vi "Generate Random Filename.vi"() -> (0 "Random Filename":string)   [LabVIEW 2022 SP3]
doc: "This VI generates a random filename. The random filename is to be used as a temporary filename, while the new VI or CTL is programmatically inserted and moved inside a LabVIEW Project, Library or Class. \n\nThe random temporary name makes it possible for the final name to be the same as another filename that already exists in the project, in a different virtual folder. (avoids name clashes)\n\nThe random filenames are sequences of 16 random lowercase characters. This makes filename clashes virtually impossible. There are 26 letters in the English alphabet, sp there are 26^16 possible 16-letter sequences.\n\nPerformance: This VI is inlined to increase performance"
uses:
  ASCII Character Type.ctl
  Generate Random ASCII Character.vi
  <vilib>/numeric/Random Number (Range).vi
  <vilib>/numeric/Random Number (Range) U64.vi
  <vilib>/numeric/sub_Random U32.vi
panel:
  # "Development\ncontrols/indicators useful for development and testing, but which are not outputs of the VI"
  # "Input\nInputs to the VI"
  # "Output\nOutputs of the VI"
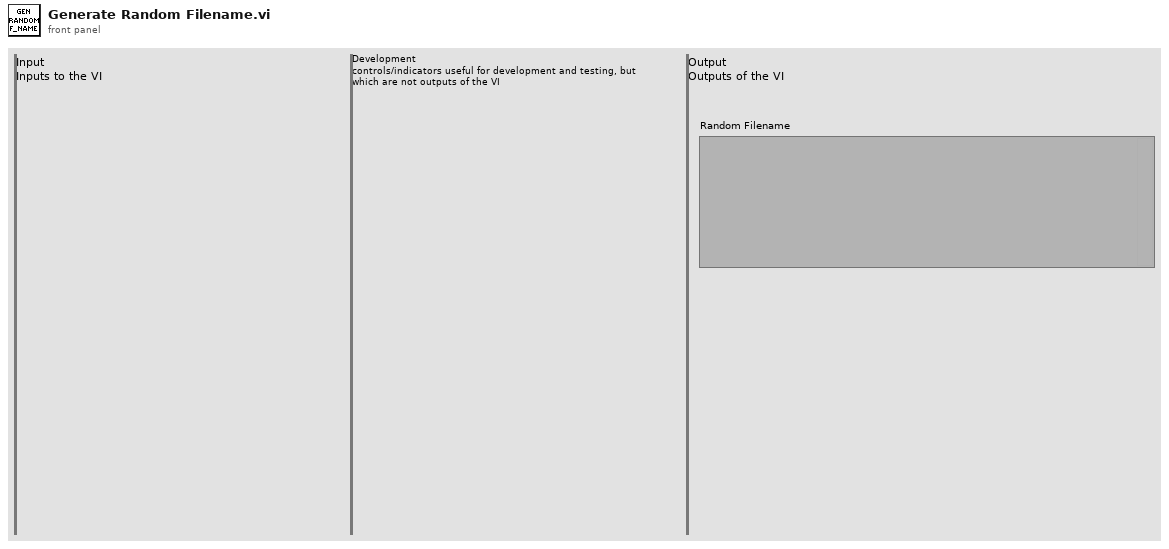
[diagram p1: front panel]
types:
  T1 = typedef "ASCII Character Type.ctl" = enum16{"Lowercase Letter", "Uppercase Letter", "Digit", "Alphanumeric", "Printable Character", "Any ASCII Character [0x00 to 0xFF]"}
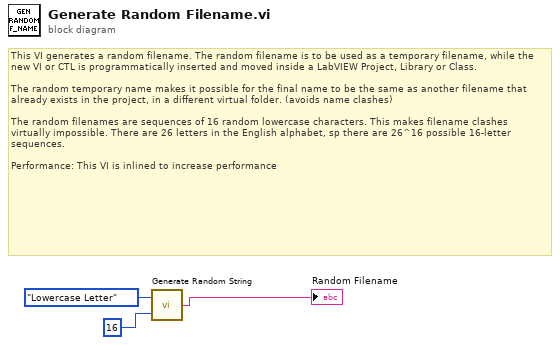
[diagram p0: block diagram]
diagram:
  # "This VI generates a random filename. The random filename is to be used as a temporary filename, while the new VI or CTL is programmatically inserted and moved inside a LabVIEW Project, Library or Class. \n\nThe random temporary name makes it possible for the final name to be the same as another filename that already exists in the project, in a different virtual folder. (avoids name clashes)\n\nThe random filenames are sequences of 16 random lowercase characters. This makes filename clashes virtually impossible. There are 26 letters in the English alphabet, sp there are 26^16 possible 16-letter sequences.\n\nPerformance: This VI is inlined to increase performance"
  n1 = call "Generate Random String.vi"("String Length (Default = 10)"=u32 16, "ASCII Character Type"=ASCII_Character_Type."Lowercase Letter") -> ("Random String"=→"Random Filename":string)
